vi "Launcher_PLC.vi"(8 "error in (no error)":errorcluster, 11 "PLC_Module in":refnum<class "PLC_Module.lvclass">) -> (0 "error out":errorcluster, 3 "PLC_Module out":refnum<class "PLC_Module.lvclass">)   [LabVIEW 2025, in "PLC_Module.lvlib" / "PLC_Module.lvclass"]
uses:
  PLC_Module.lvclass
  C:/Program Files (x86)/National Instruments/LabVIEW 2025/vi.lib/ActorFramework/Actor/Actor.lvclass
  PLC_Module.lvclass/PLC_Module.ctl
  PLC_Driver/Simulated_PLC/Simulated_PLC.lvclass
  D:/Hardware/PLC/PLC_Abstr/PLC_Abstr/PLC_Abstr.lvclass
  PLC_Driver/SIMATIC_S7/SIMATIC_S7.lvclass
  Write Connect.vi
  PLC_Abstr/PLC_Abstr/PLC_Abstr.lvclass
  <vilib>/ActorFramework/Actor/Actor.lvclass
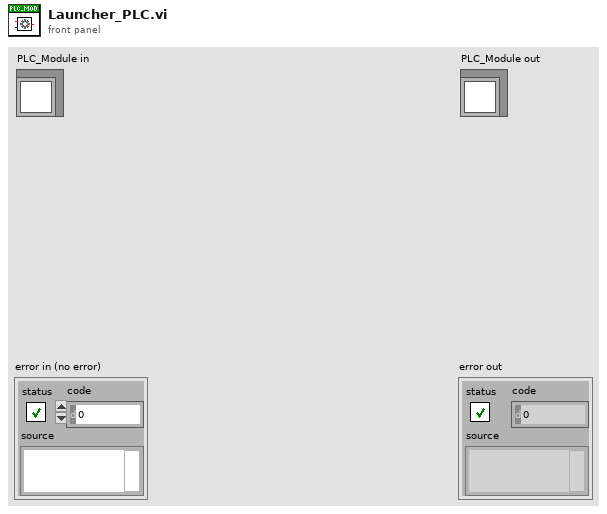
[diagram p1: front panel]
types:
  T1 = typedef "PLC_Module.lvlib/PLC_Module.lvclass/PLC_Type.ctl" = enum16{"Simulated_PLC", "SIMATIC_S7"}
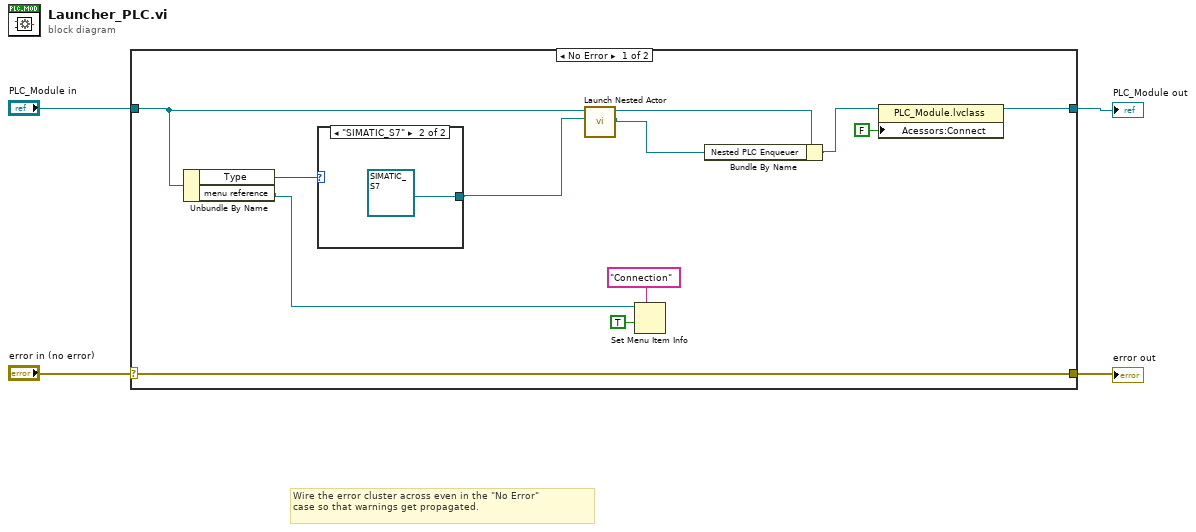
[diagram p0: block diagram]
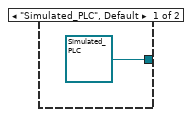
[diagram p2: hidden frame]
diagram:
  # "Wire the error cluster across even in the \"No Error\"\ncase so that warnings get propagated."
  n1 = case shown="No Error" "error in (no error)" {
    selector: "error in (no error)" -> [w16 w20]
    tunnel: [w16 w20] -> w3
    tunnel: [w9 w19] -> w1
    tunnel: "PLC_Module in" -> [w12 w19]
    frame No Error {
      n2 = Unbundle By Name(w12) -> ("Type"=w11:T1, "menu reference"=w7:refnum<k9>)
      n3 = case shown="\"SIMATIC_S7\"" w11 {
        tunnel: [refnum<class "Simulated_PLC.lvclass"> refnum ("Simulated_PLC.lvclass") refnum<class "SIMATIC_S7.lvclass"> refnum ("SIMATIC_S7.lvclass")] -> w10
        frame "Simulated_PLC", Default {
        }
        frame "SIMATIC_S7" {
        }
      }
      n4 = call <vilib>:"Launch Nested Actor.vi"("Nested Actor"=w10, "Caller Actor in"=w12) -> ("Nested Actor's Enqueuer"=w14:refnum<class "Message Enqueuer.lvclass">, "Caller Actor out"=w15:refnum<class "PLC_Module.lvclass">)  [unwired: 7 in, 1 out]
      n5 = Set Menu Item Info(7:"Connection" ("item tag"), 9:TRUE ("enabled"), 11:w7) -> ()  [unwired: 4 in, 2 out]
      n6 = Bundle By Name(cluster=w15, "Nested PLC Enqueuer"=w14) -> (w13:refnum<class "PLC_Module.lvclass">)
      n7 = property class="PLC_Module.lvclass"(reference=w13, "Acessors:Connect"=FALSE ("Connect")) -> (reference out=w9:refnum<class "PLC_Module.lvclass">)  [unwired: 1 in, 1 out]
    }
    frame Error {
    }
  }
  "error out" <- w3
  "PLC_Module out" <- w1
